vi "setPropertyStringValue.vi"(8 "error in (no error)":errorcluster, 9 "Property Value in":string, 10 "Property Name in":string, 11 "IPropertyObject in":refnum<class "IPropertyObject.lvclass">) -> (0 "error out":errorcluster, 1 "Property Value out":string, 2 "Property Name out":string, 3 "IPropertyObject out":refnum<class "IPropertyObject.lvclass">)   [LabVIEW 2022 SP3, in "openDAQ.lvlib" / "IBaseObject.lvlib" / "IPropertyObject.lvlib" / "IPropertyObject.lvclass"]
uses:
  <instrlib>/openDAQ/Public/Classes/IPropertyObject/IPropertyObject.lvclass
  C:/Program Files (x86)/National Instruments/LabVIEW 2022/instr.lib/openDAQ/Public/Classes/IBaseObject/IBaseObject.lvclass
  <instrlib>/openDAQ/Public/Classes/IBaseObject/IBaseObject.lvclass/IBaseObject.ctl
  <instrlib>/openDAQ/Public/Classes/IBaseObject/Accessor/Read reference.vi
  <instrlib>/openDAQ/Public/Classes/IBaseObject/Accessor/Write reference.vi
  <instrlib>/openDAQ/Public/Classes/daqCoreTypes/IString/IString.lvclass
  <instrlib>/openDAQ/Binaries/Windows/x86/copendaq32.dll
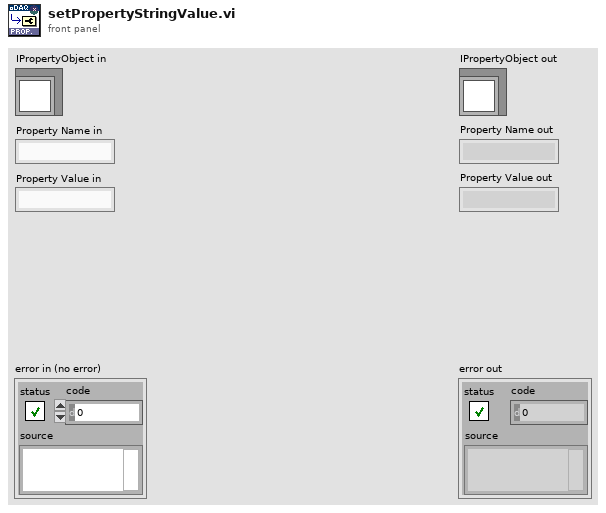
[diagram p1: front panel]
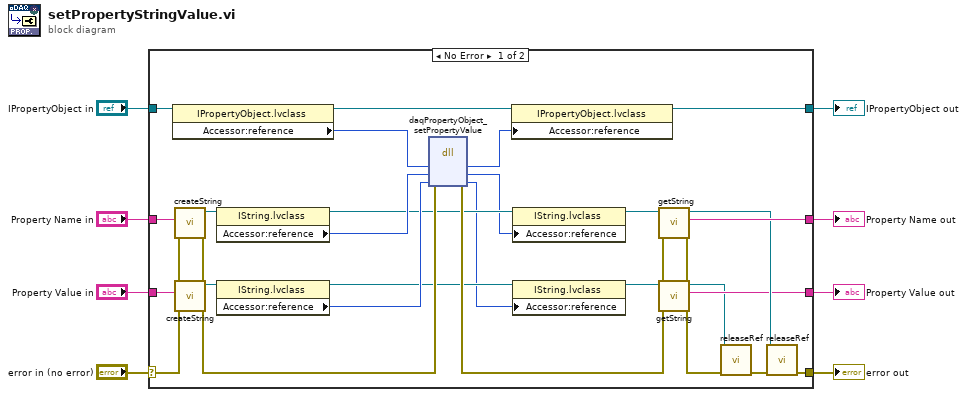
[diagram p0: block diagram]
diagram:
  n1 = case shown="No Error" "error in (no error)" {
    selector: "error in (no error)" -> [w16 w41]
    tunnel: [w23 w41] -> w7
    tunnel: [w31 w40] -> w5
    tunnel: "IPropertyObject in" -> [w34 w40]
    tunnel: "Property Name in" -> [w29 w39]
    tunnel: [w24 w39] -> w3
    tunnel: "Property Value in" -> [w17 w38]
    tunnel: [w13 w38] -> w1
    frame No Error {
      n2 = property class="IPropertyObject.lvclass"(reference=w34) -> (reference out=w32:refnum<class "IPropertyObject.lvclass">, "Accessor:reference"=w33:i64)  [unwired: 1 in, 1 out]
      n3 = call <instrlib>:"createString.vi"("error in (no error)"=w16, "String"=w17) -> ("error out"=w15:errorcluster, "IString out"=w18:refnum<class "IString.lvclass">)  [unwired: 8 in]
      n4 = call <instrlib>:"createString.vi"("error in (no error)"=w15, "String"=w29) -> ("error out"=w36:errorcluster, "IString out"=w28:refnum<class "IString.lvclass">)  [unwired: 8 in]
      n5 = property class="IString.lvclass"(reference=w28) -> (reference out=w26:refnum<class "IString.lvclass">, "Accessor:reference"=w27:i64)  [unwired: 1 in, 1 out]
      n6 = property class="IString.lvclass"(reference=w18) -> (reference out=w19:refnum<class "IString.lvclass">, "Accessor:reference"=w35:i64)  [unwired: 1 in, 1 out]
      n7 = dll-call lib="C:/Program Files (x86)/National Instruments/LabVIEW 2022/instr.lib/openDAQ/Binaries/Windows/x86/copendaq*.*" fn="daqPropertyObject_setPropertyValue"(error in=w36, "config"=w33, "propertyName"=w27, "value"=w35) -> (error out=w37:errorcluster, "config"=w30:i64, "propertyName"=w21:i64, "value"=w9:i64)  [unwired: 3 in, 1 out]
      n8 = property class="IPropertyObject.lvclass"(reference=w32, "Accessor:reference"=w30) -> (reference out=w31:refnum<class "IPropertyObject.lvclass">)  [unwired: 1 in, 1 out]
      n9 = property class="IString.lvclass"(reference=w26, "Accessor:reference"=w21) -> (reference out=w25:refnum<class "IString.lvclass">)  [unwired: 1 in, 1 out]
      n10 = property class="IString.lvclass"(reference=w19, "Accessor:reference"=w9) -> (reference out=w20:refnum<class "IString.lvclass">)  [unwired: 1 in, 1 out]
      n11 = call <instrlib>:"getString.vi"("error in (no error)"=w37, "IString in"=w20) -> ("error out"=w14:errorcluster, "String out"=w13:string, "IString out"=w10:refnum<class "IString.lvclass">)  [unwired: 7 in]
      n12 = call <instrlib>:"getString.vi"("error in (no error)"=w14, "IString in"=w25) -> ("error out"=w12:errorcluster, "String out"=w24:string, "IString out"=w22:refnum<class "IString.lvclass">)  [unwired: 7 in]
      n13 = call-dynamic "releaseRef.vi"("error in (no error)"=w12, "IBaseObject in"=w10) -> ("error out"=w11:errorcluster)  [unwired: 9 in]
      n14 = call-dynamic "releaseRef.vi"("error in (no error)"=w11, "IBaseObject in"=w22) -> ("error out"=w23:errorcluster)  [unwired: 9 in]
    }
    frame Error {
    }
  }
  "error out" <- w7
  "IPropertyObject out" <- w5
  "Property Name out" <- w3
  "Property Value out" <- w1
